vi "rmad waveform to file.vi"(6 "node name":string, 7 "event_datadir":string, 8 "error in (no error)":errorcluster, 10 "ID":u16, 11 "waveform dataset":waveform(dbl)[](array[waveform])) -> (0 "error out":errorcluster)   [LabVIEW 2017]
uses:
  <vilib>/Waveform/WDTFileIO.llb/Export Waveforms To Spreadsheet File (1D).vi
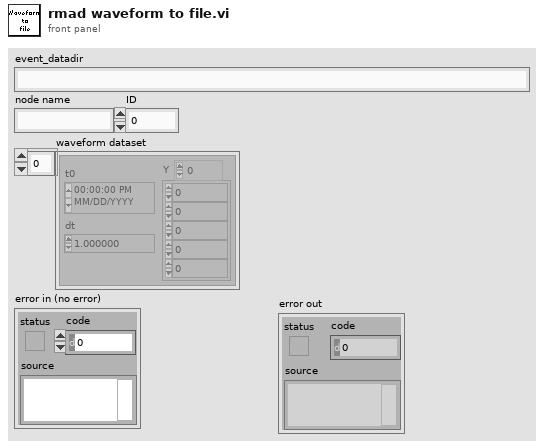
[diagram p1: front panel]
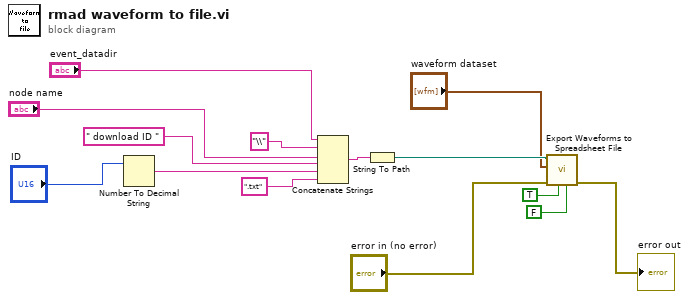
[diagram p0: block diagram]
diagram:
  n1 = Number To Decimal String(number="ID") -> (decimal integer string=w11:string)  [unwired: 1 in]
  n2 = Concatenate Strings("event_datadir", "\\" ("string"), "node name", " download ID " ("string"), w11, ".txt" ("string")) -> (w14:string)
  n3 = String To Path(string=w14) -> (path=w4:path)
  n4 = call-poly <vilib>:"Export Waveforms to Spreadsheet File.vi"("header? (write header:T)"=FALSE, "append to file? (new file:F)"=TRUE, "error in (no error)"="error in (no error)", "waveforms"="waveform dataset", "file path (dialog if empty)"=w4) -> ("error out"=→"error out":errorcluster)  [unwired: 5 in, 1 out]
